vi "Talk to Client.vi"(6 "connection ID":refnum<k5>, 8 "Error In":errorcluster, 10 "Self Enqueuer":refnum<class "Message Enqueuer.lvclass">) -> (0 "Error Out":errorcluster)   [LabVIEW 2019, in "TCP Communications.lvclass"]
uses:
  TCP Communications.lvclass
  <vilib>/ActorFramework/Message Enqueuer/Message Enqueuer.lvclass
  Communications Messages/Client Message Msg/Client Message Msg.lvclass/Client Message Msg.ctl
  <vilib>/ActorFramework/Message Enqueuer/Message Enqueuer.lvclass/Message Enqueuer.ctl
  <vilib>/ActorFramework/Message Enqueuer/Enqueue.vi
  Communications Messages/Client Message Msg/Client Message Msg.lvclass
  C:/Program Files/National Instruments/LabVIEW 2019/vi.lib/ActorFramework/Message/Message.lvclass
  <vilib>/ActorFramework/Message Priority Queue/Priority Enqueue.vi
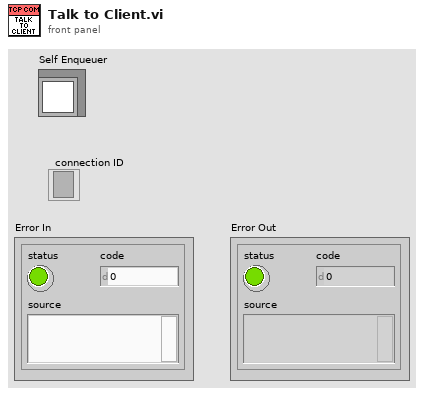
[diagram p1: front panel]
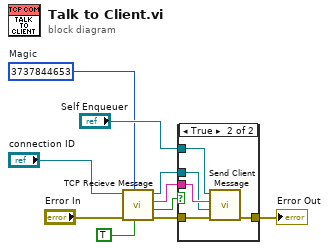
[diagram p0: block diagram]
diagram:
  w1 = u32 3737844653  # Magic
  n1 = call "TCP Recieve Message.vi"("Close on error"=TRUE, "Magic"=w1, "Error In"="Error In", "connection ID"="connection ID") -> ("Error Out"=w5:errorcluster, "Valid"=w2:bool, "Response"=w4:string, "connection ID out"=w3:refnum<k5>)  [unwired: 4 in]
  n2 = case shown="True" w2 {
    tunnel: w5 -> [w11 w14]
    tunnel: "Self Enqueuer" -> [_ w16]
    tunnel: [w11 w15] -> w9
    tunnel: w4 -> [_ w13]
    tunnel: w3 -> [_ w12]
    frame False {
    }
    frame True {
      n3 = call "Send Client Message.vi"("error in (no error)"=w14, "Context"=w12, "Message"=w13, "Message Enqueuer"=w16) -> ("error out"=w15:errorcluster)  [unwired: 6 in, 1 out]
    }
  }
  "Error Out" <- w9
